vi "ZMC Make Zar And Down2.vi"(6 "uid":u32, 7 "pPass":string, 8 "error in (no error)":errorcluster caption="错误输入（无错误）", 9 "pBasDir":string, 10 "pzpj":u32, 11 "handle":u32) -> (0 "error out":errorcluster caption="错误输出", 1 "function return":i32, 2 "pzpj out":u32, 3 "handle out":u32)   [LabVIEW 2015, in "zauxdll.lvlib"]
doc: "int32 __stdcall ZMC_MakeZarAndDown2(ZMC_HANDLE handle, void *pzpj,const char *pBasDir,const char *pPass, uint32 uid);"
uses:
  zauxdll.lvlib
  zmotion.dll
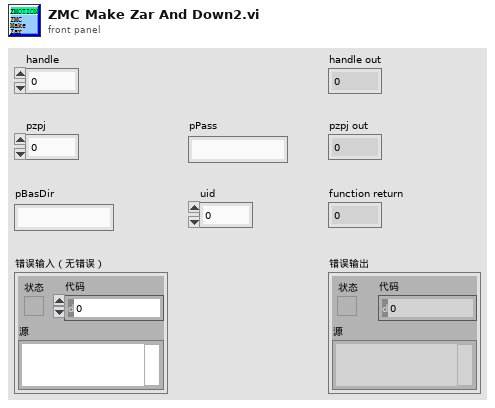
[diagram p1: front panel]
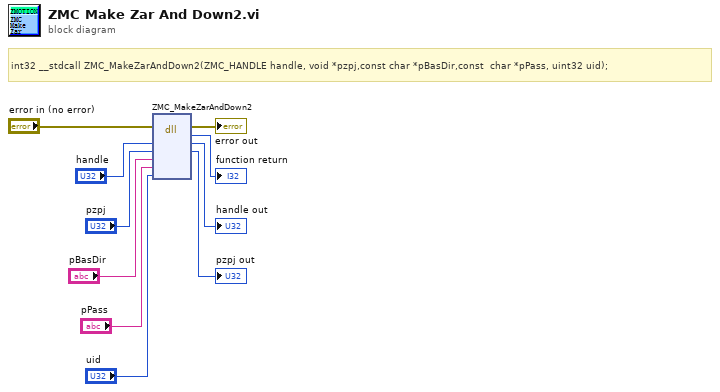
[diagram p0: block diagram]
diagram:
  # "int32 __stdcall ZMC_MakeZarAndDown2(ZMC_HANDLE handle, void *pzpj,const char *pBasDir,const  char *pPass, uint32 uid);"
  n1 = dll-call lib="C:/Users/VIC/Desktop/GOGORO_SA/system/LLB/zmotion/zaux/zmotion.*" fn="ZMC_MakeZarAndDown2"(error in="error in (no error)", "handle"="handle", "pzpj"="pzpj", "pBasDir"="pBasDir", "pPass"="pPass", "uid"="uid") -> (error out=→"error out":errorcluster, →"function return":i32, "handle"=→"handle out":u32, "pzpj"=→"pzpj out":u32)  [unwired: 5 in, 1 out]
